vi "Read.vi"(4 "Remote Path":string, 5 "Username":string, 6 "Password":string, 7 "Address":string, 8 "Error In":errorcluster) -> (0 "Error Out":errorcluster)   [LabVIEW 2017, in "Tests.lvlib" / "SFTP File.lvlib"]
uses:
  SFTP File.lvlib
  <vilib>/addons/_JKI Toolkits/Caraya/classes/Test/Test.lvclass
  <vilib>/addons/_JKI Toolkits/Caraya/classes/Assert/Assert.lvclass
  src/Toolkit/API/SFTP File/SFTP File.lvclass
  Tests.lvlib
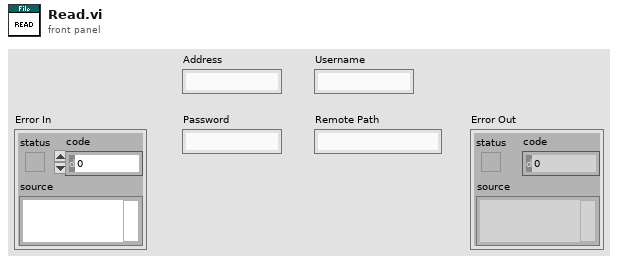
[diagram p1: front panel]
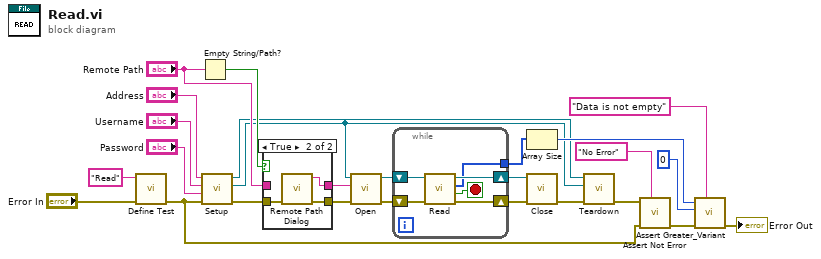
[diagram p0: block diagram]
diagram:
  n1 = call <vilib>:"Define Test.vi"("error in (no error)"="Error In", "Label (VI Title)"="Read") -> ("error out"=w6:errorcluster)  [unwired: 9 in]
  n2 = Empty String/Path?(string/path="Remote Path") -> (empty?=w22:bool)
  n3 = call "Setup.vi"("Error In"=w6, "Password"="Password", "Username"="Username", "Address"="Address") -> ("Error Out"=w5:errorcluster, "SFTP"=w1:refnum<class "SFTP.lvclass">, "Sesssion"=w2:refnum<class "Session.lvclass">)  [unwired: 5 in]
  n4 = case shown="True" w22 {
    tunnel: [w27 w31] -> w21
    tunnel: [w28 w30] -> w19
    tunnel: "Remote Path" -> [w28 _]
    tunnel: w5 -> [w27 w29]
    frame False {
    }
    frame True {
      n5 = call "Remote Path Dialog.vi"("Error In"=w29) -> ("Error Out"=w31:errorcluster, "Remote Path Out"=w30:string)  [unwired: 9 in]
    }
  }
  n6 = call "Open.vi"("Error In"=w21, "Remote Path"=w19, "SFTP"=w1) -> ("Error Out"=w17:errorcluster, "SFTP File"=w18:refnum<class "SFTP File.lvclass">)  [unwired: 7 in]
  n7 = while {
    shift-right: [w35] -> w16
    shift-left: w18 -> [w37]
    shift-right: [w34] -> w15
    shift-left: w17 -> [w36]
    tunnel: [w32] -> w14
    stop <- w33 stop-if-true
    n8 = call "Read.vi"("Error In"=w36, "SFTP File In"=w37) -> ("Error Out"=w34:errorcluster, "End-of-File?"=w33:bool, "Data"=w32:u8[], "SFTP File Out"=w35:refnum<class "SFTP File.lvclass">)  [unwired: 6 in]
  }
  n9 = Array Size(array=w14) -> (size(s)=w12:i32)
  n10 = call "Close.vi"("Error In"=w15, "SFTP"=w16) -> ("Error Out"=w4:errorcluster)  [unwired: 8 in, 1 out]
  n11 = call "Teardown.vi"("Error In"=w4, "SFTP"=w1, "Session"=w2) -> ("Error Out"=w3:errorcluster)  [unwired: 8 in]
  n12 = call <vilib>:"Assert Not Error.vi"("Label"="No Error", "error in (no error)"=w6, "Not Error?"=w3) -> ("error out"=w23:errorcluster)  [unwired: 8 in]
  n13 = call <vilib>:"Assert Greater_Variant.vi"("Label"="Data is not empty", "error in (no error)"=w23, "Y"=0 ("size(s)"), "X"=w12) -> ("error out"=→"Error Out":errorcluster)  [unwired: 7 in]
